vi "get Log Files Directory.vi"() -> (3 "Log Files Directory":path)   [LabVIEW 2015, in "System Config.lvclass"]
uses:
  System Config.lvclass
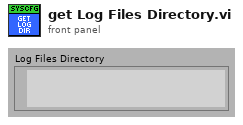
[diagram p1: front panel]
types:
  T1 = typedef "System Config.lvclass/ClassAttributes.ctl" = cluster{"Config":cluster{"Logging":cluster{"Log Files Directory":path, "Max Lines Per Log File":i32}, "Settings":T2}, "Core":cluster{"Config Directory":path, "Name":string, "Config Changed":refnum<user-event>}}
  T2 = typedef "System Config.lvclass/Settings.ctl" = cluster{"Dummy":dbl}
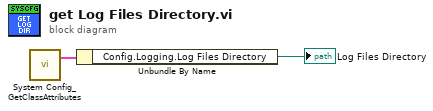
[diagram p0: block diagram]
diagram:
  n1 = call "System Config_GetClassAttributes.vi"() -> ("class attributes"=w1:T1)  [unwired: 8 in, 3 out]
  n2 = Unbundle By Name(w1) -> ("Config.Logging.Log Files Directory"=→"Log Files Directory":path)
